vi "Main.vi"() -> ()   [LabVIEW 2021]
uses:
  <vilib>/Platform/TimedLoop/XDataNode/wakeup.ctl
  <vilib>/Platform/TimedLoop/XDataNode/nitl_modes.ctl
  <vilib>/Platform/TimedLoop/XDataNode/timing_clust.ctl
  <vilib>/platform/TimedLoop/XDataNode/XDataNode.xnode
  Sub VIs/GNSS/GNSS Data.ctl
  Sub VIs/Steering Motor Encoder/Steering Motor Encoder Data.ctl
  Sub VIs/IMU/IMU Data.ctl
  Sub VIs/State Estimator/Measurements.ctl
  Sub VIs/Logging/Log Level.ctl
  Sub VIs/Steering Motor/Steering Motor Data.ctl
  Sub VIs/Drive Motor/Drive Motor Data.ctl
  Sub VIs/Logging/Controller Data.ctl
  Sub VIs/State Estimator/State Estimate.ctl
  Sub VIs/Trajectory Control/Trajectory_Control.ctl
  Sub VIs/Steering Motor/Steering Motor Handle.ctl
  <vilib>/Utility/RT CPU Load.ctl
panel:
  out "iso data out":string
  out "iso connection ID":refnum<k5>
  out "error out":errorcluster
  in  "iso adress":string
  in  "iso port":u16
  in  "error in (no error)":errorcluster
  in  "Abort Trajectory":bool
  in  "Kp":dbl
  in  "Ki":dbl
  out "Speed":bool
  in  "?":bool
  out "RPM":bool
  in  "Drive Motor Speed (m/s)":dbl
  in  "file path (trajectorymat)":path=path "c:/ni-rt/startup/trajectorymat_asta0_line.csv"
  in  "file path (matrixmat)":path=path "c:/ni-rt/startup/matrixmat_default.csv"
  out "velocity":dbl(graph)
  out "CPU loads":T1[](array[typedef]) {"ISR (%)" format="%#.2f"; "Idle (%)" format="%#.2f"; "Background (%)" format="%#.2f"; "Normal (%)" format="%#.2f"; "Above Normal (%)" format="%#.2f"; "High (%)" format="%#.2g"; "Timed Structures (%)" format="%#.2g"; "Time Critical (%)" format="%#.2g"; "Total (%)" format="%#.2g"}
  out "Measurements (Debug)":T2 {"GNSS Data"."Longitude (deg)" format="%#.10g"; "GNSS Data"."Latitude (deg)" format="%#.10g"; "GNSS Data"."Longitude (rad)" format="%#_10g"; "GNSS Data"."Latitude (rad)" format="%#_10g"}
  out "State Estimate (Debug)":T6 {"Y (m)" format="%#_10g"; "X (m)" format="%#_10g"}
  out "Motor Controllers (Debug)":T7
  out "Trajectory (Debug)":T10
  out "State estimator Ts check":bool
  out "E2 limit hit":bool
  out "E1 limit hit":bool
  out "XY trajectory (0 is bikeposition)":T11(graph)
  out "Y-Offset":dbl
  out "X-Offset":dbl
  in  "Reset and Init trajectory":bool
  in  "Drive Motor Angular Speed (rad/s)":dbl
  in  "Enable Steering Motor":bool
  out "Steering Motor Enabled":bool
  out "Abort":bool
  in  "Reset Steering Motor Encoder":bool
  in  "Stop Button":bool
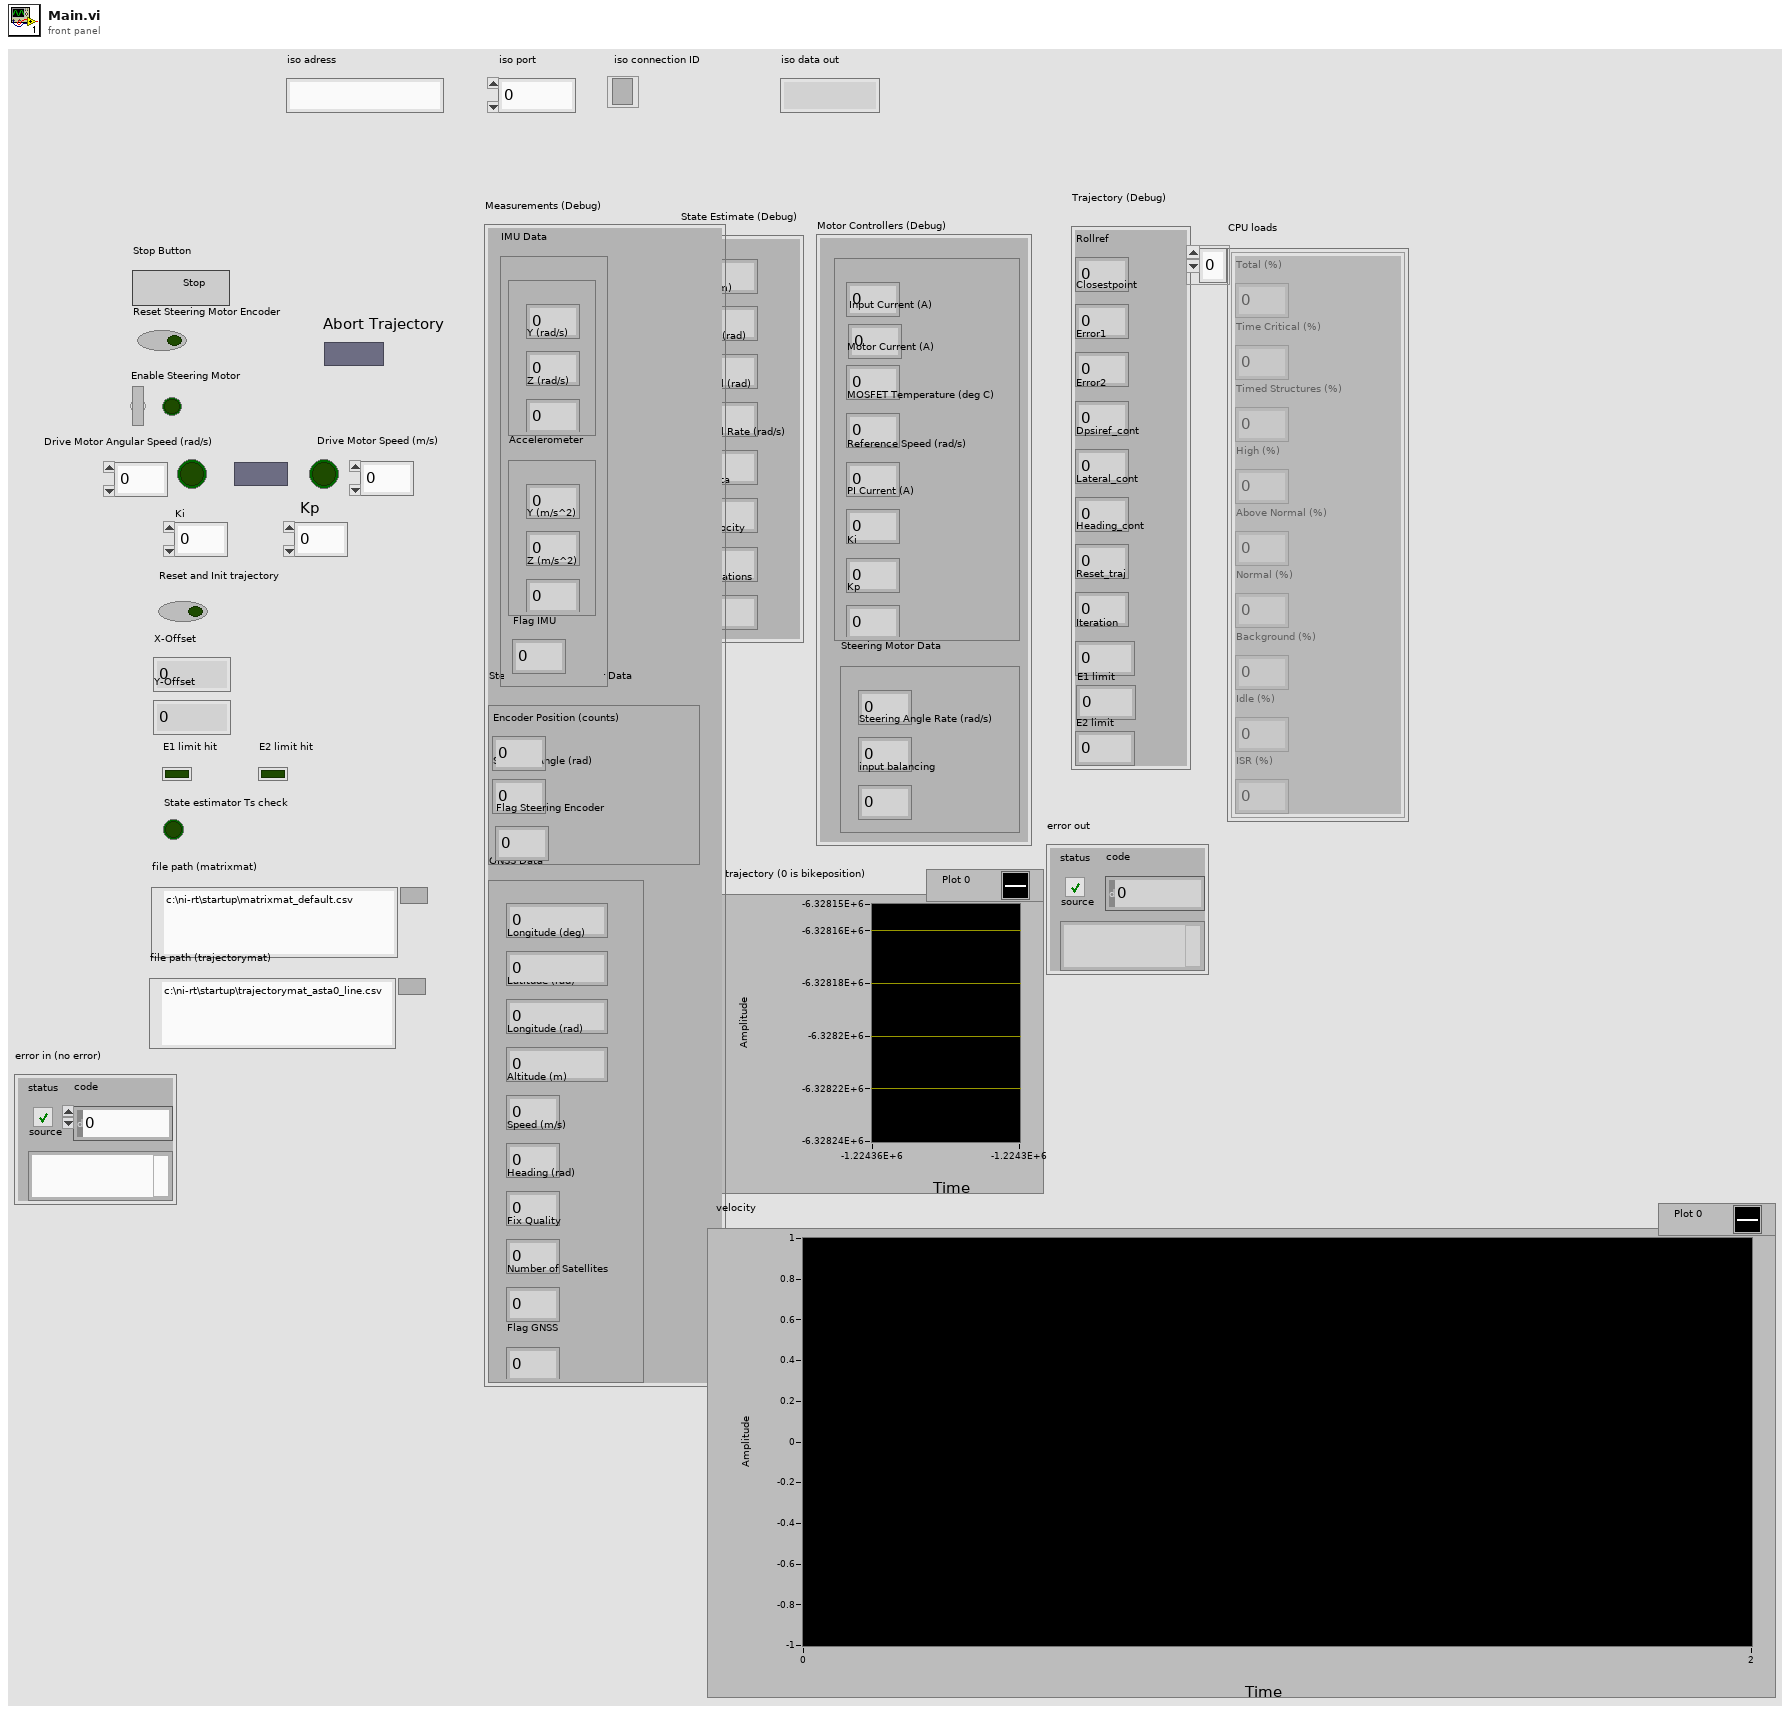
[diagram p1: front panel]
types:
  T1 = typedef "NI_Real-Time Target Support.lvlib/RT CPU Load.ctl" = cluster{"Total (%)":dbl, "Time Critical (%)":dbl, "Timed Structures (%)":dbl, "High (%)":dbl, "Above Normal (%)":dbl, "Normal (%)":dbl, "Background (%)":dbl, "Idle (%)":dbl, "ISR (%)":dbl}
  T2 = typedef "Measurements.ctl" = cluster{"IMU Data":T3, "Steering Motor Encoder Data":T4, "GNSS Data":T5}
  T3 = typedef "IMU Data.ctl" = cluster{"Gyroscope":cluster{"X (rad/s)":dbl, "Y (rad/s)":dbl, "Z (rad/s)":dbl}, "Accelerometer":cluster{"X (m/s^2)":dbl, "Y (m/s^2)":dbl, "Z (m/s^2)":dbl}, "Flag IMU":dbl}
  T4 = typedef "Steering Motor Encoder Data.ctl" = cluster{"Encoder Position (counts)":i32, "Steering Angle (rad)":dbl, "Flag Steering Encoder":dbl}
  T5 = typedef "GNSS Data.ctl" = cluster{"Latitude (rad)":dbl, "Longitude (rad)":dbl, "Altitude (m)":dbl, "Speed (m/s)":dbl, "Heading (rad)":dbl, "Fix Quality":i32, "Number of Satellites":i32, "Latitude (deg)":dbl, "Longitude (deg)":dbl, "Flag GNSS":dbl}
  T6 = typedef "State Estimate.ctl" = cluster{"X (m)":dbl, "Y (m)":dbl, "Psi (rad)":dbl, "Roll (rad)":dbl, "Roll Rate (rad/s)":dbl, "delta":dbl, "velocity":dbl, "Iterations":dbl}
  T7 = typedef "Controller Data.ctl" = cluster{"Drive Motor Data":T8, "Steering Motor Data":T9}
  T8 = typedef "Drive Motor Data.ctl" = cluster{"Angular Speed (rad/s)":dbl, "Input Current (A)":dbl, "Motor Current (A)":dbl, "MOSFET Temperature (deg C)":dbl, "Reference Speed (rad/s)":dbl, "PI Current (A)":dbl, "Ki":dbl, "Kp":dbl}
  T9 = typedef "Steering Motor Data.ctl" = cluster{"PWM":dbl, "Steering Angle Rate (rad/s)":dbl, "input balancing":dbl}
  T10 = typedef "Trajectory_Control.ctl" = cluster{"Rollref":dbl, "Closestpoint":dbl, "Error1":dbl, "Error2":dbl, "Dpsiref_cont":dbl, "Lateral_cont":dbl, "Heading_cont":dbl, "Reset_traj":dbl, "Iteration":dbl, "E1 limit":u32, "E2 limit":u32}
  T11 = cluster{"Trajectory(X/Y/PSI)":dbl[], "Trajectory(X/Y/PSI)":dbl[]}
  T12 = cluster{"Steering Angle Rate":dbl, "rollReference":dbl, "roll":dbl, "rollRate":dbl, "Kp":dbl, "Kd":dbl, "steering_flag":i32}
  T13 = typedef "XDNodeRunTimeDep.lvlib/timing_clust.ctl" = cluster{"Expected End [f-1]":u64, "Actual End [f-1]":u64, "Finished Late? [f-1]":bool, "Expected End [i-1]":u64, "Actual End [i-1]":u64, "Finished Late? [i-1]":bool, "Expected Start [i]":u64, "Actual Start [i]":u64, "Expected Start [f]":u64, "Actual Start [f]":u64, "Source Name":string, "Structure Name":string, "Period":i64, "Deadline":i64, "Offset":i64, "Start":i64, "Priority":i32, "Timeout":i32, "Mode":T14, "Wakeup Reason":T15, "Error":errorcluster, "Source Type":string, "Secondary Source Type":string, "Global End Time":u64, "Global Start Time":u64, "Frame Duration":u64, "Iteration Duration":u64, "Assigned CPU":i32, "I/O Scan Engine Mode":u32}
  T14 = typedef "XDNodeRunTimeDep.lvlib/nitl_modes.ctl" = enum32{"No Change", "Process missed periods, maintain original phase", "Discard missed periods, maintain original phase", "Process missed periods, ignore original phase", "Discard missed periods, ignore original phase"}
  T15 = typedef "XDNodeRunTimeDep.lvlib/wakeup.ctl" = enum32{"Normal", "Aborted", "Asynchronous wakeup", "Timing source error", "Timed loop error", "Timeout"}
  T16 = typedef "Steering Motor Handle.ctl" = cluster{"Dummy":dbl}
  T17 = typedef "Log Level.ctl" = enum16{"Error", "Warning", "Info"}
  T18 = cluster{"B":dbl[], "A":dbl[][], "C":dbl[][], "D":dbl[], "K":dbl[][], "Trajectory":dbl[][], "Init":dbl[], "parameter":dbl[][]}
  T19 = typedef "Configuration.ctl" = cluster{"Accelerometer Bias":cluster{"X (m/s)":dbl, "Y (m/s)":dbl, "Z (m/s)":dbl}, "Gyroscope Bias":cluster{"X (m/s)":dbl, "Y (m/s)":dbl, "Z (m/s)":dbl}, "Steering Motor Gear Ratio":dbl, "Steering Pully Gear Ratio":dbl, "Steering Encoder CPR":dbl, "Steering Motor Max RPM":dbl, "Wheelbase (m)":dbl, "Fork Angle (rad)":dbl, "Balancing Controller":cluster{"Kp (/s)":dbl, "Kd (1)":dbl}, "Max Allowed Steering Angle (rad)":dbl, "Task Periods":cluster{"Emergency Stop (us)":i64, "IMU (us)":i64, "Steering Motor Encoder (us)":i64, "State Estimator (us)":i64, "Balancing Controller (us)":i64, "GNSS (us)":i64, "Logging (us)":i64, "Drive Motor (us)":i64, "Visualization (us)":i64}, "Drive Motor Gear Ratio":dbl, "lr":dbl, "lf":dbl, "lambda":dbl, "k1":dbl, "k2":dbl, "e1_max":dbl, "Ad_t":dbl, "Bd_t":dbl, "C_t":dbl, "D_t":dbl, "Wheel radius":dbl}
  T20 = typedef "NI_Matrix.lvlib/RealMatrix.ctl" = dbl[][]
  T21 = typedef "IMU Handle.ctl" = cluster{"I2C address":u8}
  T22 = typedef "GNSS Handle.ctl" = cluster{"VISA Resource Name":refnum<visa-resource-name>}
  T23 = typedef "Drive Motor Handle.ctl" = cluster{"VISA Resource Name":refnum<visa-resource-name>}
  T24 = typedef "Log Handle.ctl" = cluster{"Data File":refnum<file>, "Event File":refnum<file>}
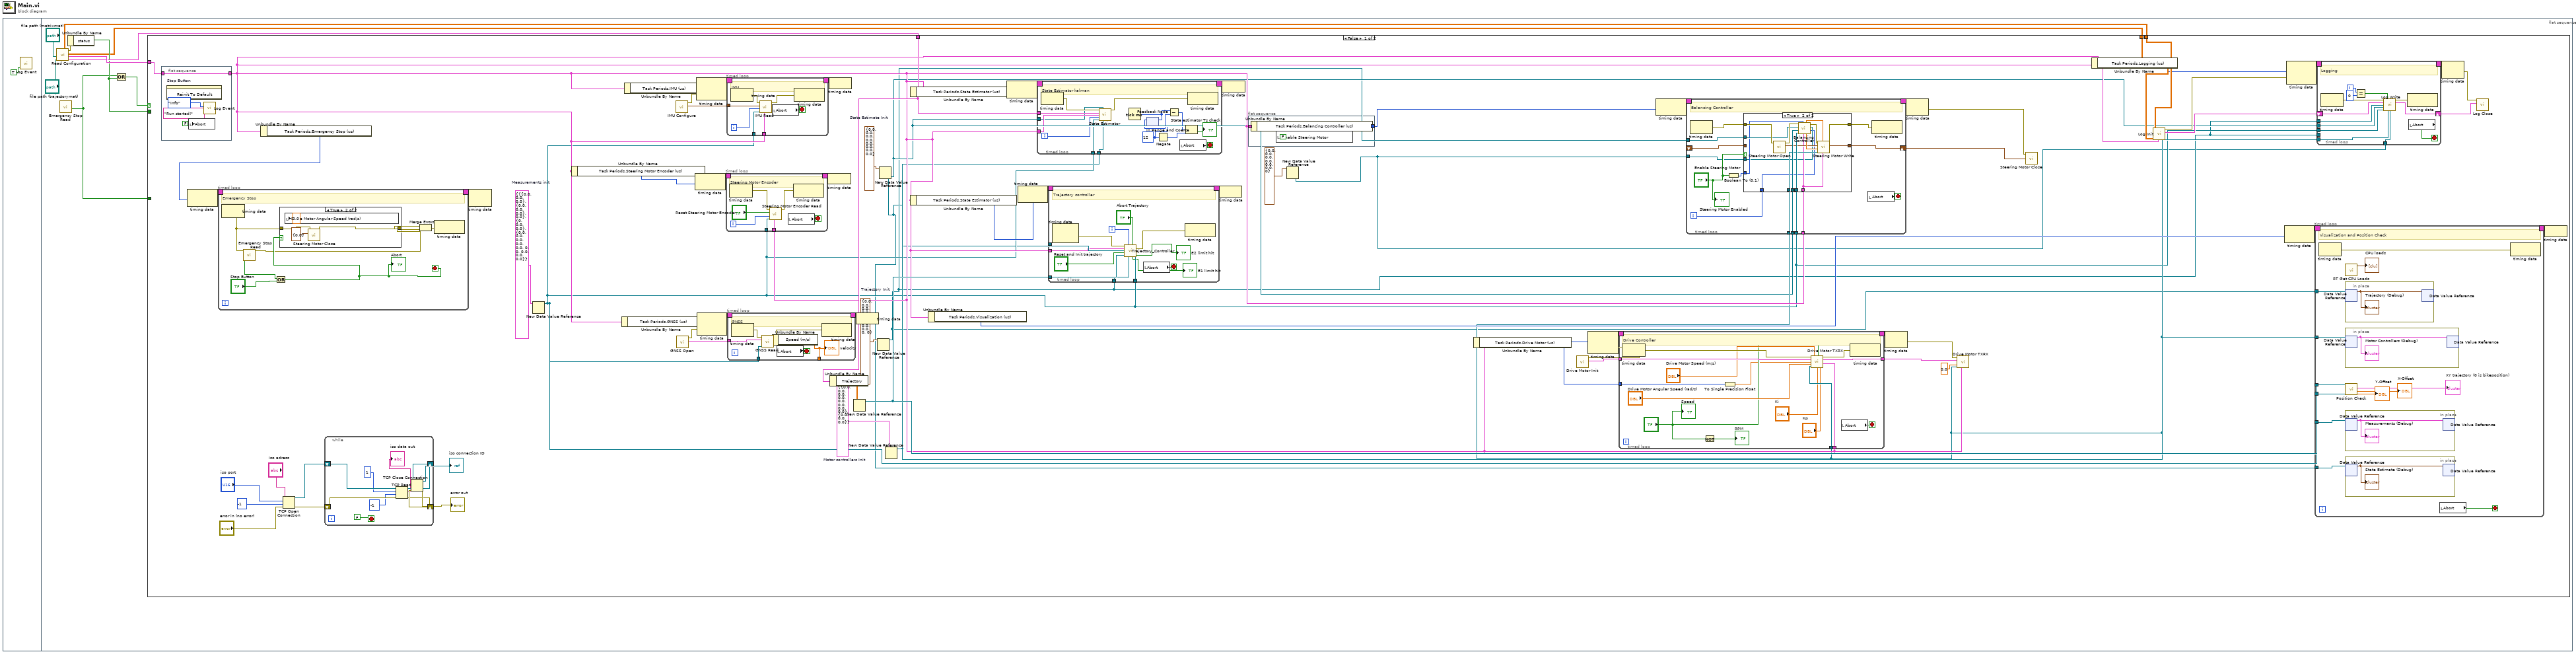
[diagram p0: block diagram]
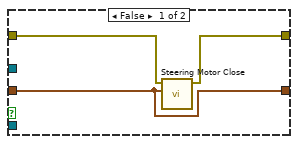
[diagram p2: hidden frame]
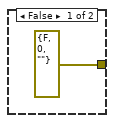
[diagram p3: hidden frame]
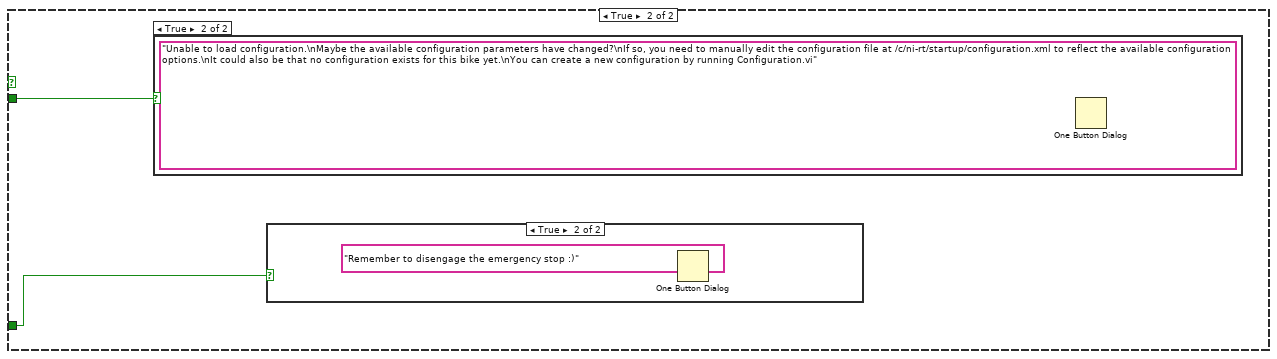
[diagram p4: hidden frame]
diagram:
  n1 = flat-sequence {
    frame #0 {
      n2 = call "Log Event.vi"("Clear Log"=TRUE) -> ()  [unwired: 10 in, 1 out]
    }
    frame #1 {
      n3 = call "Read Configuration.vi"("file path (trajectorymat)"="file path (trajectorymat)", "file path (matrixmat)"="file path (matrixmat)") -> ("values loded in xml files"=w9:T18, "configuration"=w11:T19, "value"=w4:T20, "error out"=w10:errorcluster, "Init trajectory (2)"=w6:dbl[][])  [unwired: 3 in, 2 out]
      n4 = call "Emergency Stop Read.vi"() -> ("Emergency Stop"=w7:bool)  [unwired: 10 in, 1 out]
      n5 = Unbundle By Name(w10) -> ("status"=w8:bool)
      n6 = Compound Arithmetic op=OR(w7, w8) -> (w5:bool)
      n7 = case shown="False" w5 {
        tunnel: w8 -> [_ w335]
        tunnel: w11 -> [w61 _]
        tunnel: w9 -> [w34 _]
        tunnel: w7 -> [_ w334]
        tunnel: w6 -> [w53 _]
        tunnel: w4 -> [w36 _]
        frame False {
          w42 = T10 {"Rollref"=0.0, "Closestpoint"=0.0, "Error1"=0.0, "Error2"=0.0, "Dpsiref_cont"=0.0, "Lateral_cont"=0.0, "Heading_cont"=0.0, "Reset_traj"=0.0, "Iteration"=0.0, "E1 limit"=0, "E2 limit"=0}  # Trajectory Init
          w54 = T6 {"X (m)"=0.0, "Y (m)"=0.0, "Psi (rad)"=0.0, "Roll (rad)"=0.0, "Roll Rate (rad/s)"=0.0, "delta"=0.0, "velocity"=0.0, "Iterations"=0.0}  # State Estimate Init
          w60 = T7 {"Drive Motor Data"={"Angular Speed (rad/s)"=0.0, "Input Current (A)"=0.0, "Motor Current (A)"=0.0, "MOSFET Temperature (deg C)"=0.0, "Reference Speed (rad/s)"=0.0, "PI Current (A)"=0.0, "Ki"=0.0, "Kp"=0.0}, "Steering Motor Data"={"PWM"=0.0, "Steering Angle Rate (rad/s)"=0.0, "input balancing"=0.0}}  # Motor controllers Init
          w83 = T2 {"IMU Data"={"Gyroscope"={"X (rad/s)"=0.0, "Y (rad/s)"=0.0, "Z (rad/s)"=0.0}, "Accelerometer"={"X (m/s^2)"=0.0, "Y (m/s^2)"=0.0, "Z (m/s^2)"=0.0}, "Flag IMU"=0.0}, "Steering Motor Encoder Data"={"Encoder Position (counts)"=0, "Steering Angle (rad)"=0.0, "Flag Steering Encoder"=0.0}, "GNSS Data"={"Latitude (rad)"=0.0, "Longitude (rad)"=0.0, "Altitude (m)"=0.0, "Speed (m/s)"=0.0, "Heading (rad)"=0.0, "Fix Quality"=0, "Number of Satellites"=0, "Latitude (deg)"=0.0, "Longitude (deg)"=0.0, "Flag GNSS"=0.0}}  # Measurements init
          n8 = flat-sequence {
            tunnel: [w330] -> w33
            tunnel: w61 -> [w330]
            frame #0 {
              n9 = invoke on="Stop Button" class="Bool (strict)" method="Reinit To Default"() -> ()  [unwired: 3 in, 3 out]
              n10 = local write "Abort"(FALSE ("Abort")) -> ()
              n11 = call "Log Event.vi"("Message"="Run started!", "Log Level"=Log_Level."Info") -> ()  [unwired: 9 in, 1 out]
            }
          }
          n12 = Unbundle By Name(w33) -> ("Task Periods.Emergency Stop (us)"=w82:i64)
          n13 = node-c288(w82) -> (w81:T13)
          n14 = timed-loop {
            timing: w81 -> [_]
            timing-out: [_] -> w80
            stop <- w313 stop-if-true
            # "Emergency Stop"
            n15 = node-c288() -> (w315:errorcluster)  [unwired: 1 in]
            n16 = call "Emergency Stop Read.vi"("Error In"=w315) -> ("Emergency Stop"=w310:bool, "Error Out"=w311:errorcluster)  [unwired: 9 in]
            n17 = Or(x=w310, y="Stop Button") -> (x .or. y?=w313:bool)
            "Abort" <- w313
            n18 = case shown="True" w313 {
              tunnel: w315 -> [_ w320]
              tunnel: [errorcluster {"status"=FALSE, "code"=0, "source"=""} ("Error Out") w319] -> w312
              frame False {
              }
              frame True {
                n19 = local write "Drive Motor Angular Speed (rad/s)"(0.0 ("Drive Motor Angular Speed (rad/s)")) -> ()
                n20 = call "Steering Motor Close.vi"("Steering Motor Handle"=T16 {"Dummy"=0.0}, "Error In"=w320) -> ("Error Out"=w319:errorcluster)  [unwired: 9 in]
              }
            }
            n21 = Merge Errors(w312, w311) -> (w314:errorcluster)
            n22 = node-c288(w314) -> ()  [unwired: 1 out]
          }
          n23 = TCP Open Connection(address="iso adress", remote port or service name="iso port", timeout ms (60000)=-1, error in (no error)="error in (no error)") -> (connection ID=w17:refnum<k5>, error out=w18:errorcluster)  [unwired: 1 in]
          n24 = while {
            shift-right: [w88] -> w15
            shift-left: w18 -> [w89]
            shift-right: [w87] -> w16
            shift-left: w17 -> [w90]
            stop <- FALSE stop-if-true
            n25 = TCP Read(connection ID=w90, bytes to read=1, error in (no error)=w89, 9:-1 ("timeout ms (25000)")) -> (connection ID out=w87:refnum<k5>, data out=→"iso data out":string, error out=w88:errorcluster)  [unwired: 1 in]
          }
          n26 = TCP Close Connection(connection ID=w16, error in (no error)=w15) -> (connection ID out=→"iso connection ID":refnum<k5>, error out=→"error out":errorcluster)  [unwired: 1 in]
          n27 = node-c288(w80) -> ()  [unwired: 1 out]
          n28 = New Data Value Reference(data value=w83) -> (data value reference=w29:refnum<data-value>)  [unwired: 1 in, 1 out]
          n29 = Unbundle By Name(w33) -> ("Task Periods.Steering Motor Encoder (us)"=w66:i64)
          n30 = Unbundle By Name(w33) -> ("Task Periods.GNSS (us)"=w63:i64)
          n31 = Unbundle By Name(w33) -> ("Task Periods.IMU (us)"=w67:i64)
          n32 = call "IMU Configure.vi"() -> ("IMU Handle"=w68:T21, "Error Out"=w69:errorcluster)  [unwired: 10 in]
          n33 = call "GNSS Open.vi"() -> ("GNSS Handle"=w64:T22, "Error Out"=w65:errorcluster)  [unwired: 10 in]
          n34 = node-c288(w66) -> (w73:T13)
          n35 = node-c288(w67, w69) -> (w75:T13)
          n36 = node-c288(w63, w65) -> (w71:T13)
          n37 = timed-loop {
            timing: w73 -> [_]
            timing-out: [_] -> w72
            tunnel: w29 -> [w232]
            tunnel: w33 -> [w230]
            i -> [w231]
            stop <- w233 stop-if-true
            # "Steering Motor Encoder"
            n38 = node-c288() -> (w236:errorcluster)  [unwired: 1 in]
            n39 = call "Steering Motor Encoder Read.vi"("Configuration"=w230, "Measurement In"=w232, "Flag Steering Encoder"=w231, "Reset Counter"="Reset Steering Motor Encoder", "Error In"=w236) -> ("Error Out"=w235:errorcluster)  [unwired: 4 in, 2 out]
            n40 = local read "Abort"() -> (w233:bool)
            n41 = node-c288(w235) -> ()  [unwired: 1 out]
          }
          n42 = timed-loop {
            timing: w75 -> [_]
            timing-out: [_] -> w74
            tunnel: w68 -> [w250]
            tunnel: w29 -> [w248]
            tunnel: w33 -> [w247]
            i -> [w246]
            stop <- w249 stop-if-true
            # "IMU"
            n43 = node-c288() -> (w252:errorcluster)  [unwired: 1 in]
            n44 = call "IMU Read.vi"("Configuration"=w247, "Measurement In"=w248, "Flag IMU"=w246, "IMU Handle"=w250, "Error In"=w252) -> ("Error Out"=w251:errorcluster)  [unwired: 4 in, 2 out]
            n45 = local read "Abort"() -> (w249:bool)
            n46 = node-c288(w251) -> ()  [unwired: 1 out]
          }
          n47 = timed-loop {
            timing: w71 -> [_]
            timing-out: [_] -> w70
            tunnel: w64 -> [w219]
            tunnel: w29 -> [w215]
            tunnel: [w213] -> _
            stop <- w216 stop-if-true
            # "GNSS"
            n48 = node-c288() -> (w218:errorcluster)  [unwired: 1 in]
            n49 = call "GNSS Read.vi"("Measurement In"=w215, "GNSS Handle"=w219, "Error In"=w218) -> ("GNSS Data"=w214:T5, "Error Out"=w217:errorcluster)  [unwired: 6 in, 1 out]
            n50 = Unbundle By Name(w214) -> ("Speed (m/s)"=w213:dbl)
            "velocity" <- w213
            n51 = local read "Abort"() -> (w216:bool)
            n52 = node-c288(w217) -> ()  [unwired: 1 out]
          }
          n53 = node-c288(w72) -> ()
          n54 = node-c288(w74) -> ()
          n55 = Unbundle By Name(w34) -> ("Trajectory"=w41:dbl[][])
          n56 = New Data Value Reference(data value=w41) -> (data value reference=w35:refnum<data-value>)  [unwired: 1 in, 1 out]
          n57 = node-c288(w70) -> ()
          n58 = New Data Value Reference(data value=w42) -> (data value reference=w27:refnum<data-value>)  [unwired: 1 in, 1 out]
          n59 = New Data Value Reference(data value=w54) -> (data value reference=w28:refnum<data-value>)  [unwired: 1 in, 1 out]
          n60 = New Data Value Reference(data value=w60) -> (data value reference=w30:refnum<data-value>)  [unwired: 1 in, 1 out]
          n61 = Unbundle By Name(w33) -> ("Task Periods.State Estimator (us)"=w31:i64)
          n62 = Unbundle By Name(w33) -> ("Task Periods.State Estimator (us)"=w43:i64)
          n63 = Unbundle By Name(w33) -> ("Task Periods.Visualization (us)"=w37:i64)
          n64 = node-c288(w31) -> (w45:T13)
          n65 = node-c288(w43) -> (w23:T13)
          n66 = timed-loop {
            timing: w45 -> [_]
            timing-out: [_] -> w44
            tunnel: w29 -> [w147]
            tunnel: w34 -> [w150]
            tunnel: w30 -> [w146]
            tunnel: w28 -> [w145]
            tunnel: w33 -> [w149]
            i -> [w148]
            stop <- w153 stop-if-true
            w139 = i64 12 ("y")
            # "State Estimator kalman"
            n67 = node-c288() -> (w152:errorcluster)  [unwired: 1 in]
            n68 = call "State Estimator.vi"("Error In"=w152, "State Estimate In"=w145, "Matrix"=w150, "Configuration"=w149, "Iteration"=w148, "Measurement In"=w147, "Balancing controller In"=w146) -> ("Error out"=w151:errorcluster)  [unwired: 7 in, 1 out]
            n69 = Tick Count (ms)() -> (millisecond timer value=w144:u32)
            n70 = feedback-in #1(w144) -> ()
            n71 = feedback #1() -> (w143:u32)  [unwired: 1 in]
            n72 = Negate(x=w139) -> (-x=w140:i64)
            n73 = Subtract(x=w144, y=w143) -> (x-y=w141:u32)
            n74 = local read "Abort"() -> (w153:bool)
            n75 = In Range and Coerce(upper limit=w139, x=w141, lower limit=w140) -> (In Range?=→"State estimator Ts check":bool)  [unwired: 1 out]
            n76 = node-c288(w151) -> ()  [unwired: 1 out]
          }
          n77 = timed-loop {
            timing: w23 -> [_]
            timing-out: [_] -> w22
            tunnel: w28 -> [w103]
            tunnel: w33 -> [w100]
            tunnel: w29 -> [w98]
            tunnel: w35 -> [w97]
            tunnel: w27 -> [w95]
            i -> [w99]
            stop <- w104 stop-if-true
            # "Trajectory controller"
            n78 = node-c288() -> (w101:errorcluster)  [unwired: 1 in, 1 out]
            n79 = call "Trajectory_Controller.vi"("Error In"=w101, "reset"=w99, "Abort Trajectory"="Abort Trajectory", "Configuration"=w100, "State Estimate In"=w103, "Reset and Init trajectory"="Reset and Init trajectory", "RefTraj in"=w97, "Trajectory In"=w95, "Measurement In"=w98) -> ("Error out"=w102:errorcluster, "E1 limit"=→"E1 limit hit":bool, "E2 limit"=→"E2 limit hit":bool)  [unwired: 2 in, 2 out]
            n80 = local read "Abort"() -> (w104:bool)
            n81 = node-c288(w102) -> ()  [unwired: 1 out]
          }
          n82 = node-c288(w22) -> ()
          n83 = node-c288(w44) -> ()
          n84 = flat-sequence {
            tunnel: [w264] -> w62
            tunnel: w33 -> [w263]
            frame #0 {
              n85 = Unbundle By Name(w263) -> ("Task Periods.Balancing Controller (us)"=w264:i64)
              n86 = local write "Enable Steering Motor"(FALSE ("Enable Steering Motor")) -> ()
            }
          }
          n87 = New Data Value Reference(data value=T12 {"Steering Angle Rate"=0.0, "rollReference"=0.0, "roll"=0.0, "rollRate"=0.0, "Kp"=0.0, "Kd"=0.0, "steering_flag"=0} ("output cluster")) -> (data value reference=w25:refnum<data-value>)  [unwired: 1 in, 1 out]
          n88 = Unbundle By Name(w33) -> ("Task Periods.Drive Motor (us)"=w24:i64)
          n89 = call "Drive Motor Init.vi"() -> ("Drive Motor Handle"=w50:T23, "Error Out"=w49:errorcluster)  [unwired: 10 in]
          n90 = node-c288(w24, w49) -> (w52:T13)
          n91 = timed-loop {
            timing: w52 -> [_]
            timing-out: [_] -> w51
            tunnel: w50 -> [w175]
            tunnel: w33 -> [w171]
            tunnel: w30 -> [w172]
            tunnel: [w176] -> w46
            tunnel: w24 -> [w163]
            stop <- w177 stop-if-true
            # "Drive Controller"
            n92 = node-c288() -> (w174:errorcluster)  [unwired: 1 in]
            n93 = Not(x="?") -> (.not. x?=→"RPM":bool)
            n94 = To Single Precision Float(number=w163) -> (single precision float=w164:sgl)
            n95 = call "Drive Motor TXRX.vi"("Error In"=w174, "Speed Control (m/s)"="Drive Motor Speed (m/s)", "RPM / Speed"="?", "Drive Motor Handle In"=w175, "Tasking Period"=w164, "RPM Control (rad/s)"="Drive Motor Angular Speed (rad/s)", "Controller Data In"=w172, 12:w171, "Ki"="Ki", "Kp"="Kp") -> ("Error Out"=w173:errorcluster, "Drive Motor Handle Out"=w176:T23)  [unwired: 2 in, 2 out]
            n96 = local read "Abort"() -> (w177:bool)
            n97 = node-c288(w173) -> ()  [unwired: 1 out]
            "Speed" <- "?"
          }
          n98 = node-c288(w62) -> (w79:T13)
          n99 = timed-loop {
            timing: w79 -> [_]
            timing-out: [_] -> w78
            tunnel: w28 -> [w275]
            tunnel: w29 -> [w274]
            shift-right: [w276] -> w77
            shift-left: _ -> [w273]
            tunnel: w33 -> [w272]
            tunnel: w30 -> [w271]
            tunnel: w27 -> [w270]
            tunnel: w25 -> [w267]
            i -> [w266]
            stop <- w279 stop-if-true
            # "Balancing Controller"
            n100 = node-c288() -> (w278:errorcluster)  [unwired: 1 in]
            n101 = Boolean To (0,1)(Boolean="Enable Steering Motor") -> (0, 1=w268:i16)
            n102 = case shown="True" "Enable Steering Motor" {
              tunnel: w278 -> [w282 w292]
              tunnel: [w281 w297] -> w277
              tunnel: [w280 w296] -> w276
              tunnel: w275 -> [_ w294]
              tunnel: w274 -> [_ w293]
              tunnel: w273 -> [w280 _]
              tunnel: w272 -> [_ w288]
              tunnel: w271 -> [_ w289]
              tunnel: w270 -> [_ w287]
              tunnel: w268 -> [_ w285]
              tunnel: w267 -> [_ w284]
              tunnel: w266 -> [_ w283]
              frame False {
                n103 = call "Steering Motor Close.vi"("Steering Motor Handle"=w280, "Error In"=w282) -> ("Error Out"=w281:errorcluster)  [unwired: 9 in]
              }
              frame True {
                n104 = call "Steering Motor Open.vi"("Error In"=w292) -> ("Steering Motor Handle"=w290:T16, "Error Out"=w291:errorcluster)  [unwired: 9 in]
                n105 = call "Balancing Controller.vi"("t"=w283, "Balance In"=w284, "Configuration"=w288, "steering indicator flag"=w285, "Measurement In"=w293, "State Estimate In"=w294, "Trajectory In"=w287, "Error In"=w291) -> ("Error Out"=w298:errorcluster, "Steering Angle Rate (rad/s)"=w295:dbl, "Input balancing"=w286:dbl)  [unwired: 1 out]
                n106 = call "Steering Motor Write.vi"("Configuration"=w288, "Input balancing"=w286, "Controller Data In"=w289, "Steering Angle Rate (rad/s)"=w295, "Steering Motor Handle In"=w290, "Error In"=w298) -> ("Steering Motor Handle Out"=w296:T16, "Error Out"=w297:errorcluster)  [unwired: 2 in, 2 out]
              }
            }
            n107 = local read "Abort"() -> (w279:bool)
            n108 = node-c288(w277) -> ()  [unwired: 1 out]
            "Steering Motor Enabled" <- "Enable Steering Motor"
          }
          n109 = node-c288(w51) -> (w48:errorcluster)
          n110 = node-c288(w78) -> (w76:errorcluster)
          n111 = call "Drive Motor TXRX.vi"("Error In"=w48, "Drive Motor Handle In"=w46, "RPM Control (rad/s)"=0.0 ("Angular Speed (rad/s)"), "Controller Data In"=w30, 12:w33) -> ()  [unwired: 7 in, 4 out]
          n112 = call "Steering Motor Close.vi"("Steering Motor Handle"=w77, "Error In"=w76) -> ()  [unwired: 9 in, 1 out]
          n113 = Unbundle By Name(w33) -> ("Task Periods.Logging (us)"=w32:i64)
          n114 = call "Log Init.vi"("Configuration"=w33, "Matrices"=w36, "Trajectory"=w53) -> ("Log Handle"=w55:T24, "Error Out"=w57:errorcluster)  [unwired: 7 in]
          n115 = node-c288(w37) -> (w39:T13)
          n116 = node-c288(w32, w57) -> (w59:T13)
          n117 = timed-loop {
            timing: w39 -> [_]
            timing-out: [_] -> w38
            tunnel: w35 -> [w124]
            tunnel: w29 -> [w123]
            tunnel: w30 -> [w119]
            tunnel: w29 -> [w118]
            tunnel: w28 -> [w117]
            tunnel: w27 -> [w116]
            stop <- w114 stop-if-true
            # "Visualization and Position Check"
            n118 = node-c288() -> (w125:errorcluster)  [unwired: 1 in]
            n119 = call <vilib>:"RT Get CPU Loads.vi"() -> ("CPU loads"=→"CPU loads":T1[])  [unwired: 10 in, 1 out]
            n120 = in-place {
              n121 = in-place-dvr #2(w116) -> (w126:T10)  [unwired: 1 out]
              "Trajectory (Debug)" <- w126
              n122 = in-place-dvr #2(w126) -> ()  [unwired: 2 out]
            }
            n123 = in-place {
              n124 = in-place-dvr #3(w119) -> (w127:T7)  [unwired: 1 out]
              "Motor Controllers (Debug)" <- w127
              n125 = in-place-dvr #3(w127) -> ()  [unwired: 2 out]
            }
            n126 = call "Position Check.vi"("data value reference 2"=w123, "data value reference"=w124) -> ("Y-Offset"=→"Y-Offset":dbl, "X-Offset"=→"X-Offset":dbl, "XY Graph"=→"XY trajectory (0 is bikeposition)":T11)  [unwired: 7 in]
            n127 = in-place {
              n128 = in-place-dvr #4(w118) -> (w129:T2)  [unwired: 1 out]
              "Measurements (Debug)" <- w129
              n129 = in-place-dvr #4(w129) -> ()  [unwired: 2 out]
            }
            n130 = in-place {
              n131 = in-place-dvr #5(w117) -> (w128:T6)  [unwired: 1 out]
              "State Estimate (Debug)" <- w128
              n132 = in-place-dvr #5(w128) -> ()  [unwired: 2 out]
            }
            n133 = local read "Abort"() -> (w114:bool)
            n134 = node-c288(w125) -> ()  [unwired: 1 out]
          }
          n135 = timed-loop {
            timing: w59 -> [_]
            timing-out: [_] -> w58
            tunnel: w29 -> [w191]
            tunnel: w28 -> [w194]
            shift-right: [w196] -> w40
            shift-left: w55 -> [w195]
            tunnel: w30 -> [w193]
            tunnel: w27 -> [w192]
            tunnel: w27 -> [_]
            tunnel: w25 -> [w189]
            i -> [w190]
            stop <- w201 stop-if-true
            # "Logging"
            n136 = node-c288() -> (w198:errorcluster)  [unwired: 1 in]
            n137 = Equal?(x=w190, y=0) -> (x = y?=w199:bool)
            n138 = call "Log Write.vi"("Error In"=w198, "Write Header"=w199, "Log Handle In"=w195, "Trajectory In"=w192, "State Estimate In"=w194, "Measurement In"=w191, "Controller Data In"=w193, "Balance In"=w189) -> ("Error Out"=w197:errorcluster, "Log Handle Out"=w196:T24)  [unwired: 1 in, 5 out]
            n139 = node-c288(w197) -> ()  [unwired: 1 out]
            n140 = local read "Abort"() -> (w201:bool)
          }
          n141 = node-c288(w58) -> (w56:errorcluster)
          n142 = call "Log Close.vi"("Log Handle In"=w40, "Error In"=w56) -> ()  [unwired: 9 in, 1 out]
          n143 = node-c288(w38) -> ()
        }
        frame True {
          n144 = case shown="True" w335 {
            frame False {
            }
            frame True {
              n145 = One Button Dialog(message="Unable to load configuration.\nMaybe the available configuration parameters have changed?\nIf so, you need to manually edit the configuration file at /c/ni-rt/startup/configuration.xml to reflect the available configuration options.\nIt could also be that no configuration exists for this bike yet.\nYou can create a new configuration by running Configuration.vi") -> ()  [unwired: 1 in, 1 out]
            }
          }
          n146 = case shown="True" w334 {
            frame False {
            }
            frame True {
              n147 = One Button Dialog(message="Remember to disengage the emergency stop :)") -> ()  [unwired: 1 in, 1 out]
            }
          }
        }
      }
    }
  }
